vi "判断调焦.vi"(0 "Arr Refnum":refnum<vi>, 9 "选项":i32 min=0 max=5 step=1, 11 "error in":errorcluster) -> (4 "垂直清晰度-数值":dbl, 6 "垂直清晰度":bool, 8 "水平清晰度-数值":dbl, 10 "水平清晰度":bool, 15 "error out":errorcluster)   [LabVIEW 2016]
uses:
  <vilib>/Analysis/baseanly.llb/Mean (DBL).vi
  <vilib>/Analysis/NI_AALBase.lvlib
panel:
  out "Value":u16[][](array[numeric])
  out "Max value":dbl
  out "Min value":dbl
  out "Y坐标":dbl
  out "X 坐标":dbl
  out "垂直Bre":dbl
  out "水平Bre":dbl
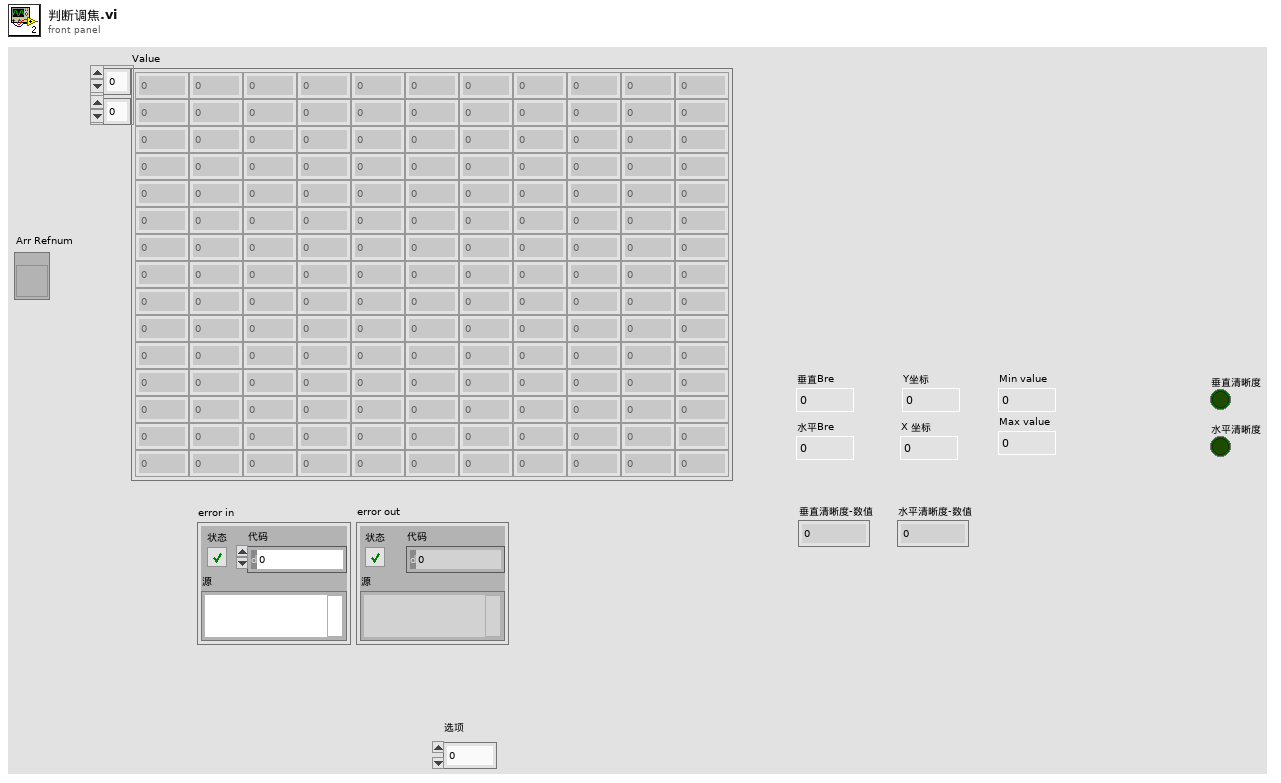
[diagram p1: front panel]
types:
  T1 = cluster{"CalData":path, "Datasave":path, "Data":path}
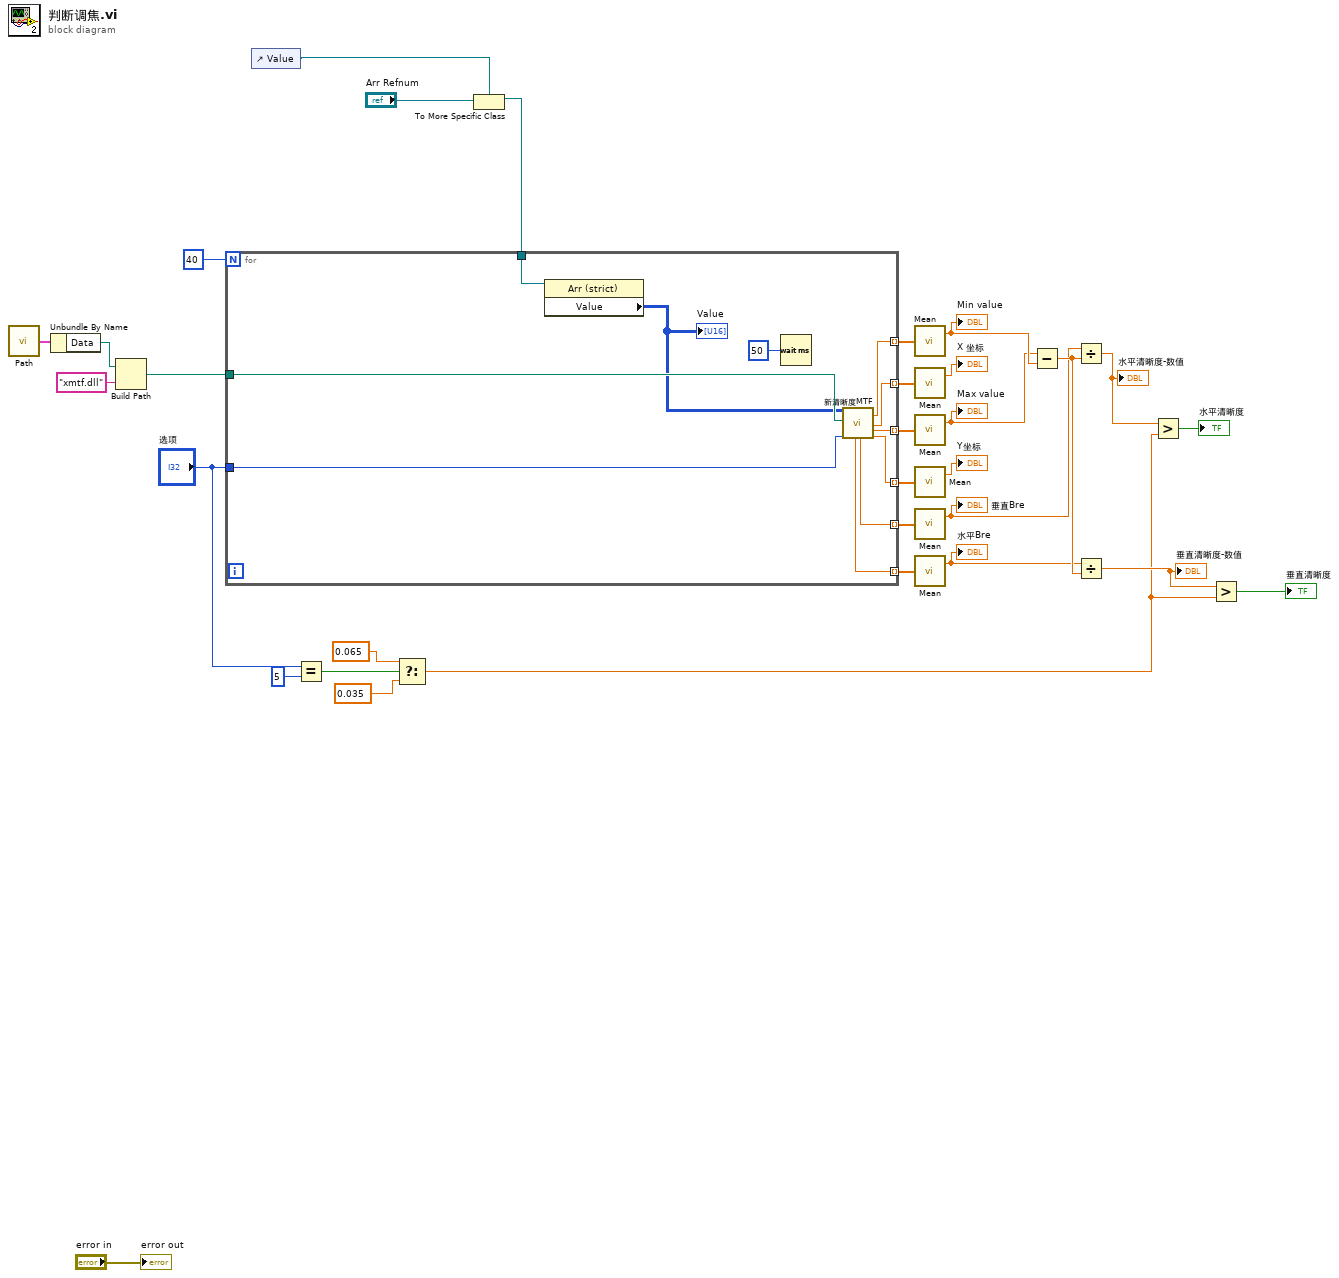
[diagram p0: block diagram]
diagram:
  n1 = call "Path.vi"() -> ("path"=w14:T1)  [unwired: 9 in]
  n2 = Unbundle By Name(w14) -> ("Data"=w12:path)
  n3 = Build Path(base path=w12, name or relative path="xmtf.dll") -> (appended path=w11:path)
  n4 = control-ref of="Value"() -> (w8:refnum<vi>)
  n5 = Equal?(x="选项", y=5) -> (x = y?=w4:bool)
  n6 = Select(t=0.065, s=w4, f=0.035) -> (s? t:f=w1:dbl)
  n7 = To More Specific Class(target class=w8, reference="Arr Refnum") -> (specific class reference=w9:refnum<vi>)  [unwired: 1 in, 1 out]
  n8 = for {
    N: 40 -> [_]
    tunnel: [w43] -> w15 mode=indexing
    tunnel: [w42] -> w20 mode=indexing
    tunnel: [w41] -> w24 mode=indexing
    tunnel: [w40] -> w18 mode=indexing
    tunnel: [w39] -> w21 mode=indexing
    tunnel: [w38] -> w25 mode=indexing
    tunnel: "选项" -> [w37]
    tunnel: w11 -> [w35]
    tunnel: w9 -> [w34]
    n9 = property class="Arr (strict)"(reference=w34) -> ("Value"=w33:u16[][])  [unwired: 1 in, 2 out]
    "Value" <- w33
    n10 = Wait (ms)(milliseconds to wait=u32 50) -> ()  [unwired: 1 out]
    n11 = call "新清晰度MTF.vi"("Image Pixels"=w33, "path in"=w35, "焦距选择"=w37) -> ("水平Bre"=w43:dbl, "垂直Bre"=w40:dbl, "Min value"=w41:dbl, "X 坐标"=w39:dbl, "Max value"=w42:dbl, "Y坐标"=w38:dbl)  [unwired: 9 in, 2 out]
  }
  n12 = call-poly <vilib>:"Mean.vi"("X"=w24) -> ("mean"=w23:dbl)  [unwired: 1 out]
  "Min value" <- w23
  n13 = call-poly <vilib>:"Mean.vi"("X"=w21) -> ("mean"=→"X 坐标":dbl)  [unwired: 1 out]
  n14 = call-poly <vilib>:"Mean.vi"("X"=w20) -> ("mean"=w19:dbl)  [unwired: 1 out]
  "Max value" <- w19
  n15 = call-poly <vilib>:"Mean.vi"("X"=w25) -> ("mean"=→"Y坐标":dbl)  [unwired: 1 out]
  n16 = call-poly <vilib>:"Mean.vi"("X"=w18) -> ("mean"=w17:dbl)  [unwired: 1 out]
  "垂直Bre" <- w17
  n17 = call-poly <vilib>:"Mean.vi"("X"=w15) -> ("mean"=w16:dbl)  [unwired: 1 out]
  "水平Bre" <- w16
  n18 = Subtract(x=w19, y=w23) -> (x-y=w29:dbl)
  n19 = Divide(x=w17, y=w29) -> (x/y=w28:dbl)
  "水平清晰度-数值" <- w28
  n20 = Divide(x=w16, y=w29) -> (x/y=w30:dbl)
  "垂直清晰度-数值" <- w30
  n21 = Greater?(x=w28, y=w1) -> (0:→"水平清晰度":bool)
  n22 = Greater?(x=w30, y=w1) -> (0:→"垂直清晰度":bool)
  "error out" <- "error in"
